vi "Задание_АБ.vi"() -> ()   [LabVIEW 2013]
panel:
  out "Массив с паузами":dbl[](array[numeric])
  in  "Количество бит":i32=8
  out "Вырезка из массива":dbl[](array[numeric])
  out "Биты на выходе 1":dbl[](array[numeric])
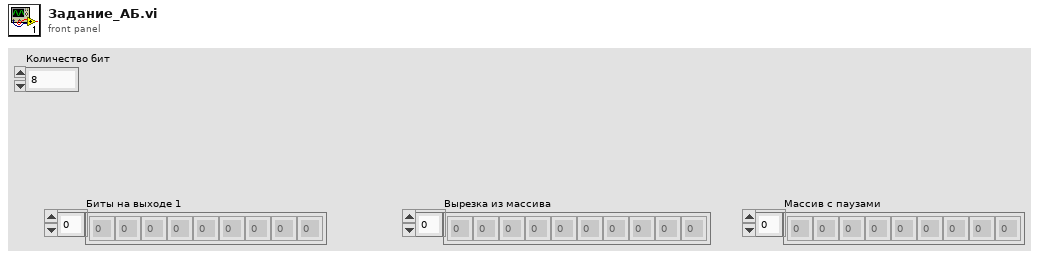
[diagram p1: front panel]
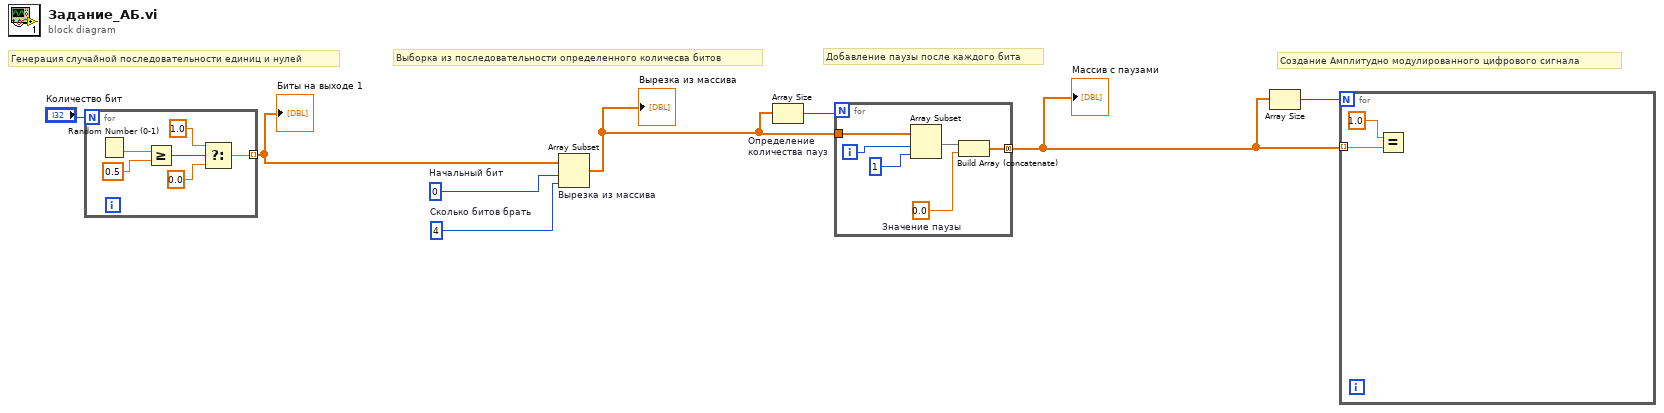
[diagram p0: block diagram]
diagram:
  w6 = 4  # Сколько битов брать
  w7 = 0  # Начальный бит
  # "Создание Амплитудно модулированного цифрового сигнала"
  # "Добавление паузы после каждого бита"
  # "Выборка из последовательности определенного количесва битов"
  # "Генерация случайной последовательности единиц и нулей"
  n1 = for {
    N: "Количество бит" -> [_]
    tunnel: [w9] -> w5 mode=indexing
    n2 = Random Number (0-1)() -> (number: 0 to 1=w14:dbl)
    n3 = Greater Or Equal?(x=w14, y=0.5) -> (x >= y?=w12:bool)
    n4 = Select(t=1.0, s=w12, f=0.0) -> (s? t:f=w9:dbl)
  }
  "Биты на выходе 1" <- w5
  n5 = Array Subset "Вырезка из массива"(array=w5, index=w7, length=w6) -> (w3:dbl[])
  "Вырезка из массива" <- w3
  n6 = Array Size "Определение количества пауз"(array=w3) -> (size(s)=w4:i32)
  n7 = for {
    N: w4 -> [_]
    tunnel: w3 -> [w17]
    tunnel: [w16] -> w1 mode=concatenating
    i -> [w15]
    w18 = 0.0  # Значение паузы
    n8 = Array Subset(array=w17, index=w15, length=1) -> (w19:dbl[])
    n9 = Build Array (concatenate)(w19, w18) -> (w16:dbl[])
  }
  "Массив с паузами" <- w1
  n10 = Array Size(array=w1) -> (size(s)=w2:i32)
  n11 = for {
    N: w2 -> [_]
    tunnel: w1 -> [w22] mode=indexing
    n12 = Equal?(x=1.0, y=w22) -> ()  [unwired: 1 out]
  }
